vi "OPM.GetPower.vi"(8 "error in (no error)":errorcluster, 11 "PM in":refnum<class "OPM.Simulated.lvclass">) -> (0 "error out":errorcluster, 2 "Power, W":dbl format="%#_13g", 3 "PM out":refnum<class "OPM.Simulated.lvclass">)   [LabVIEW 2017, in "OPM.Simulated.lvclass"]
uses:
  OPM.Simulated.lvclass
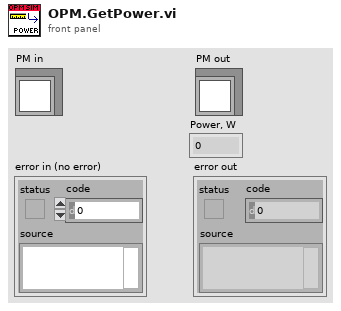
[diagram p1: front panel]
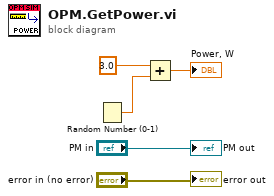
[diagram p0: block diagram]
diagram:
  n1 = Random Number (0-1)() -> (number: 0 to 1=w3:dbl)
  n2 = Add(x=3.0, y=w3) -> (x+y=→"Power, W":dbl)
  "error out" <- "error in (no error)"
  "PM out" <- "PM in"
